vi "Image_RAW12_U8_to_RAW12_U16.vi"(8 "error in (no error)":errorcluster, 11 "RAW12 Frame (U8)":u8[](array[numeric])) -> (0 "error out":errorcluster, 3 "RAW12 Frame (U16)":u16[](array[numeric]))   [LabVIEW 2020]
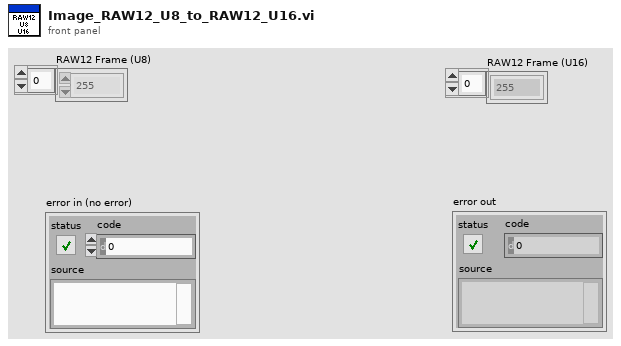
[diagram p1: front panel]
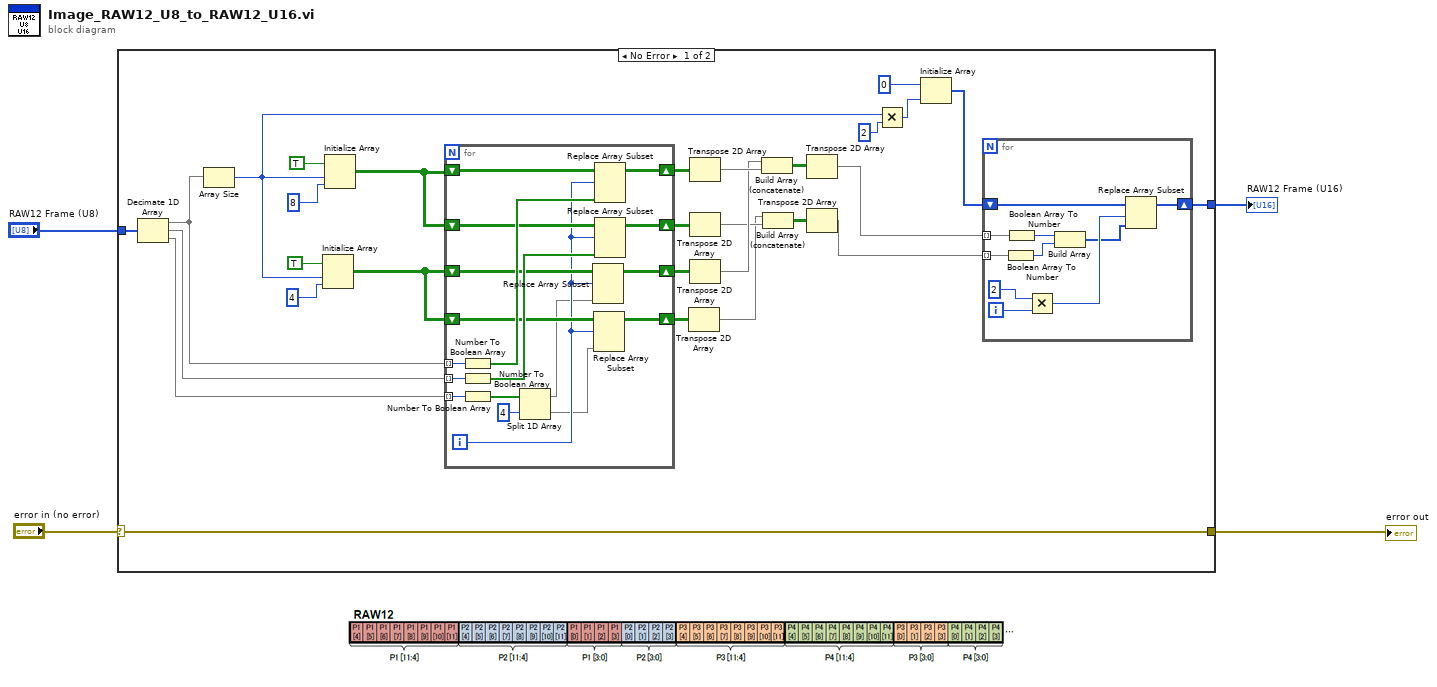
[diagram p0: block diagram]
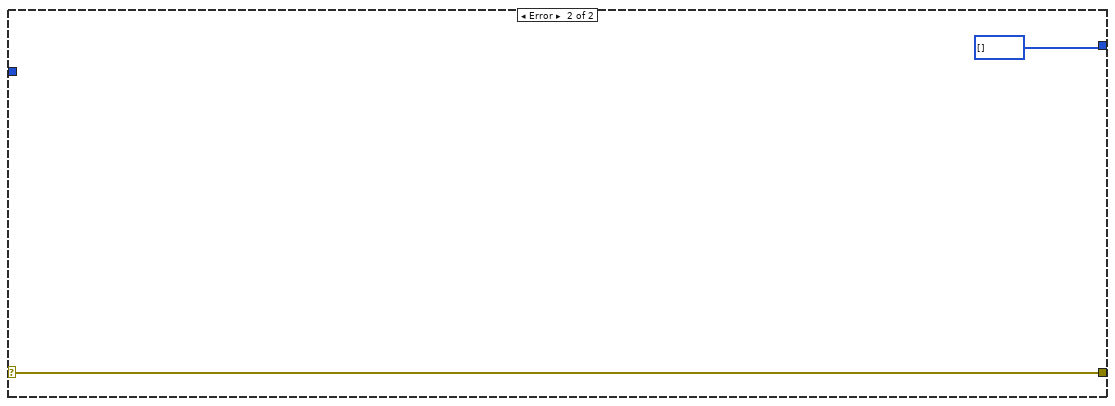
[diagram p2: hidden frame]
diagram:
  n1 = case shown="No Error" "error in (no error)" {
    selector: "error in (no error)" -> [w5 w63]
    tunnel: "RAW12 Frame (U8)" -> [w33 _]
    tunnel: [w5 w63] -> w2
    tunnel: [w6 u16[] []] -> w1
    frame No Error {
      n2 = Decimate 1D Array(w33) -> (w26:u8[], w25:u8[], w24:u8[])
      n3 = Array Size(array=w26) -> (size(s)=w10:i32)
      n4 = Initialize Array(TRUE, w10, 4 ("y")) -> (w27:bool[][])
      n5 = Initialize Array(TRUE, w10, 8 ("y")) -> (w30:bool[][])
      n6 = for {
        tunnel: w26 -> [w61] mode=indexing
        shift-right: [w58] -> w23
        shift-left: w30 -> [w60]
        shift-right: [w56] -> w22
        shift-left: w30 -> [w57]
        tunnel: w25 -> [w55] mode=indexing
        tunnel: w24 -> [w53] mode=indexing
        shift-right: [w51] -> w21
        shift-left: w27 -> [w52]
        shift-right: [w47] -> w20
        shift-left: w27 -> [w48]
        i -> [w46]
        n7 = Number To Boolean Array(number=w61) -> (Boolean array=w59:bool[])
        n8 = Number To Boolean Array(number=w55) -> (Boolean array=w54:bool[])
        n9 = Number To Boolean Array(number=w53) -> (Boolean array=w50:bool[])
        n10 = Split 1D Array(array=w50, index=4) -> (first subarray=w45:bool[], second subarray=w44:bool[])
        n11 = Replace Array Subset(array=w52, new element=w45, index (row)=w46) -> (w51:bool[][])  [unwired: 1 in]
        n12 = Replace Array Subset(array=w48, new element=w44, index (row)=w46) -> (w47:bool[][])  [unwired: 1 in]
        n13 = Replace Array Subset(array=w60, new element=w59, index (row)=w46) -> (w58:bool[][])  [unwired: 1 in]
        n14 = Replace Array Subset(array=w57, new element=w54, index (row)=w46) -> (w56:bool[][])  [unwired: 1 in]
      }
      n15 = Transpose 2D Array(2D array=w20) -> (transposed array=w16:bool[][])
      n16 = Transpose 2D Array(2D array=w23) -> (transposed array=w19:bool[][])
      n17 = Transpose 2D Array(2D array=w22) -> (transposed array=w17:bool[][])
      n18 = Transpose 2D Array(2D array=w21) -> (transposed array=w18:bool[][])
      n19 = Build Array (concatenate)(w18, w19) -> (w15:bool[][])
      n20 = Build Array (concatenate)(w16, w17) -> (w14:bool[][])
      n21 = Transpose 2D Array(2D array=w15) -> (transposed array=w9:bool[][])
      n22 = Transpose 2D Array(2D array=w14) -> (transposed array=w8:bool[][])
      n23 = Multiply(x=w10, y=2) -> (x*y=w11:i32)
      n24 = Initialize Array(u16 0, w11) -> (w7:u16[])
      n25 = for {
        tunnel: w9 -> [w43] mode=indexing
        tunnel: w8 -> [w42] mode=indexing
        shift-right: [w34] -> w6
        shift-left: w7 -> [w41]
        i -> [w38]
        n26 = Boolean Array To Number(Boolean array=w42) -> (number=w39:u16)
        n27 = Boolean Array To Number(Boolean array=w43) -> (number=w40:u16)
        n28 = Multiply(x=2, y=w38) -> (x*y=w36:i32)
        n29 = Build Array(w40, w39) -> (w35:u16[])
        n30 = Replace Array Subset(array=w41, new element=w35, index=w36) -> (w34:u16[])
      }
    }
    frame Error {
    }
  }
  "RAW12 Frame (U16)" <- w1
  "error out" <- w2
